vi "Pfeiffer Vacuum Turbo Pumping station controlling.vi"(8 "error in (no error)":errorcluster, 9 "PV Pumping station - Cluster":T1={"Parameter"=0, "Parameter\nread only<->describe"=FALSE, "Op. mode backing pump"=0, "Pmin for backing-pump\ninterval operations [W]"=40, "Config. Acces. A1 (old version)"=0, "Config. Acces. B1 (old version)"=0, "Pmax for backing-pump\ninterval operations [W]"=40} {"Pmax for backing-pump\ninterval operations [W]" min=30 max=90 step=1; "Config. Acces. B1 (old version)" items=[" fan (constant) (default)", " venting valve", " heating", " backing pump", " fan (temperature controlled)", " seal gas", " always off", " always on"]; "Config. Acces. A1 (old version)" items=[" fan (constant)", " venting valve", " heating", " backing pump", " fan (temperature controlled)", " seal gas", " always off", " always on"]; "Op. mode backing pump" items=[" non-stop", " intermittent", " switch on delayed"]; "Pmin for backing-pump\ninterval operations [W]" min=30 max=90 step=1; "Parameter" items=[" Operations mode backing pump (default)", " Configuration Accessories A1 (old version)", " Configuration Accessories B1 (old version)", " Actual pressure value  [mbar]   (read only)", " Vacuum pressure gauge type", " Pmin for backing-pump interval operations [W]", " Pmax for backing-pump interval operations [W]"]}, 10 "Adress of unit":u16=1 min=1 max=999 step=1, 11 "COM Port Name in":refnum<visa-resource-name>="COM1") -> (0 "error out":errorcluster, 3 "response (data)":string)   [LabVIEW 2021]
doc: "This VI is an example of how to use the Pfeiffer Vacuum subVIs programmatically. This VI first initializes the instrument, takes measurements, then closes the instrument."
uses:
  <instrlib>/Pfeiffer Vacuum/Public/Turbopumps/PV Pumping station - Cluster.ctl
  <instrlib>/Pfeiffer Vacuum/Pfeiffer Vacuum.lvlib
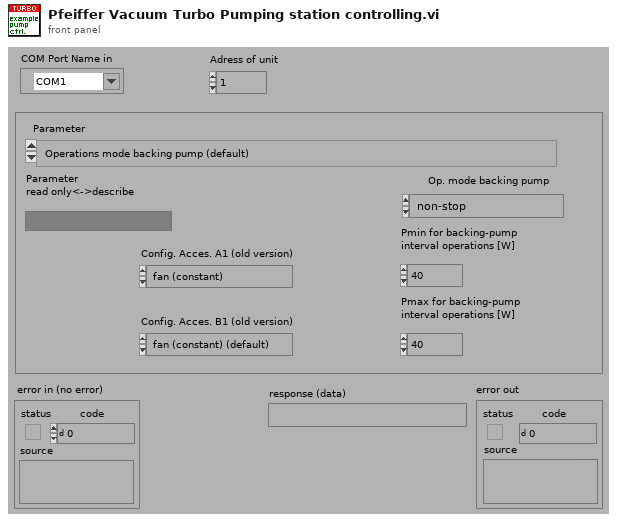
[diagram p1: front panel]
types:
  T1 = typedef "Pfeiffer Vacuum.lvlib/PV Pumping station - Cluster.ctl" = cluster{"Parameter":u16, "Parameter\nread only<->describe":bool, "Op. mode backing pump":u16, "Pmin for backing-pump\ninterval operations [W]":u16, "Config. Acces. A1 (old version)":u16, "Config. Acces. B1 (old version)":u16, "Pmax for backing-pump\ninterval operations [W]":u16}
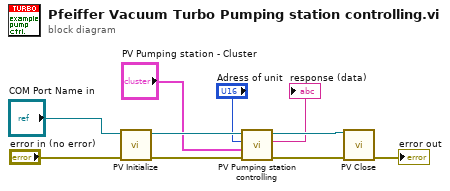
[diagram p0: block diagram]
diagram:
  n1 = call <instrlib>:"PV Initialize.vi"("error in (no error)"="error in (no error)", "VISA session in"="COM Port Name in") -> ("error out"=w10:errorcluster, "VISA session out"=w8:refnum<visa-resource-name>)  [unwired: 8 in]
  n2 = call <instrlib>:"PV Pumping station controlling.vi"("error in (no error)"=w10, "PV Pumping station - Cluster"="PV Pumping station - Cluster", "Adress of unit"="Adress of unit", "VISA session"=w8) -> ("error out"=w9:errorcluster, "response (data)"=→"response (data)":string, "dup VISA session"=w7:refnum<visa-resource-name>)  [unwired: 5 in]
  n3 = call <instrlib>:"PV Close.vi"("VISA session"=w7, "error in (no error)"=w9) -> ("error out"=→"error out":errorcluster)  [unwired: 13 in]
